vi "line_terminate.vi"(8 "error in (no error)":errorcluster, 11 "AnalysisRAPS in":refnum<class "AnalysisRAPS.lvclass">) -> (0 "error out":errorcluster, 3 "AnalysisRAPS out":refnum<class "AnalysisRAPS.lvclass">)   [LabVIEW 2010, in "AnalysisRAPS.lvclass"]
uses:
  AnalysisRAPS.lvclass
  AnalysisRAPS.lvclass/AnalysisRAPS.ctl
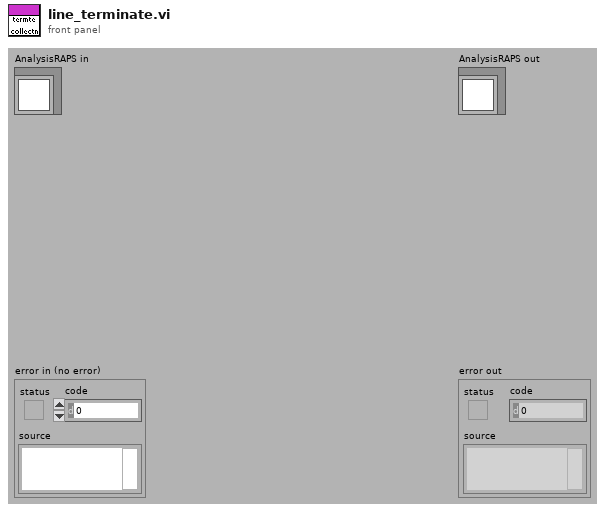
[diagram p1: front panel]
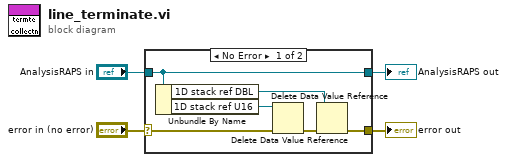
[diagram p0: block diagram]
diagram:
  n1 = case shown="No Error" "error in (no error)" {
    selector: "error in (no error)" -> [w8 w12]
    tunnel: [w6 w12] -> w3
    tunnel: [w10 w11] -> w1
    tunnel: "AnalysisRAPS in" -> [w10 w11]
    frame No Error {
      n2 = Unbundle By Name(w10) -> ("1D stack ref DBL"=w5:refnum<data-value>, "1D stack ref U16"=w9:refnum<data-value>)
      n3 = Delete Data Value Reference(data value reference=w9, error in=w8) -> (error out=w7:errorcluster)  [unwired: 1 out]
      n4 = Delete Data Value Reference(data value reference=w5, error in=w7) -> (error out=w6:errorcluster)  [unwired: 1 out]
    }
    frame Error {
    }
  }
  "error out" <- w3
  "AnalysisRAPS out" <- w1
